vi "initialize_constants.vi"(8 "error in (no error)":errorcluster) -> (0 "error out":errorcluster)   [LabVIEW 2021]
uses:
  Constants.vi
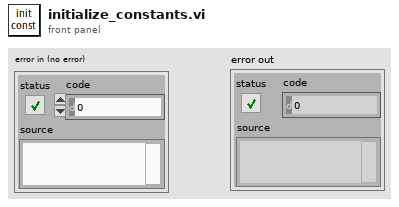
[diagram p1: front panel]
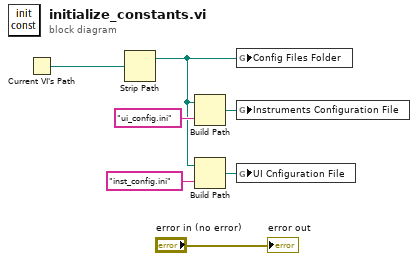
[diagram p0: block diagram]
diagram:
  n1 = Current VI's Path() -> (path=w2:path)
  n2 = Strip Path(path=w2) -> (stripped path=w1:path)  [unwired: 1 out]
  n3 = Build Path(base path=w1, name or relative path="ui_config.ini") -> (appended path=w5:path)
  n4 = Build Path(base path=w1, name or relative path="inst_config.ini") -> (appended path=w6:path)
  n5 = global write "Constants.vi" "Config Files Folder"(w1) -> ()
  n6 = global write "Constants.vi" "Instruments Configuration File"(w5) -> ()
  n7 = global write "Constants.vi" "UI Cnfiguration File"(w6) -> ()
  "error out" <- "error in (no error)"
